vi "BL_TestConnection.vi"(8 "error in (no error)":errorcluster, 11 "Potentiostat Galvanostat in":refnum<class "Potentiostat Galvanostat.lvclass">) -> (0 "error out":errorcluster, 3 "Potentiostat Galvanostat out":refnum<class "Potentiostat Galvanostat.lvclass">)   [LabVIEW 2018, in "Potentiostat Galvanostat.lvclass"]
doc: "This function tests the communication with the selected instrument."
uses:
  Potentiostat Galvanostat.lvclass
  Potentiostat Galvanostat.lvclass/Potentiostat Galvanostat.ctl
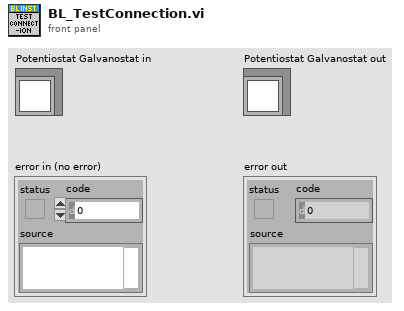
[diagram p1: front panel]
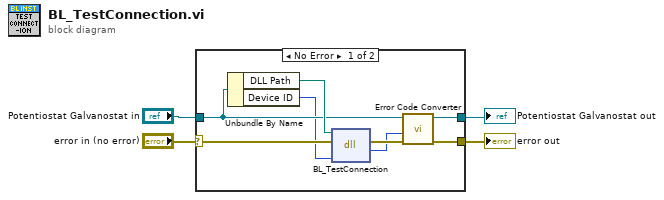
[diagram p0: block diagram]
diagram:
  n1 = case shown="No Error" "error in (no error)" {
    selector: "error in (no error)" -> [w11 w14]
    tunnel: [w9 w14] -> w3
    tunnel: [w8 w13] -> w1
    tunnel: "Potentiostat Galvanostat in" -> [w6 w13]
    frame No Error {
      n2 = Unbundle By Name(w6) -> ("DLL Path"=w12:path, "Device ID"=w5:i32)
      n3 = dll-call lib="C:/Projects/LabVIEW/BioLogic Instrument Driver/libs/EC-Lab Development Package/EClib.*" fn="BL_TestConnection"(path in=w12, error in=w11, "Device ID"=w5) -> (error out=w10:errorcluster, "Error Code"=w7:i32)  [unwired: 2 in, 1 out]
      n4 = call-dynamic "Error Code Converter.vi"("error in (no error)"=w10, "Error Code"=w7, "Potentiostat Galvanostat in"=w6) -> ("error out"=w9:errorcluster, "Potentiostat Galvanostat out"=w8:refnum<class "Potentiostat Galvanostat.lvclass">)  [unwired: 7 in]
    }
    frame Error {
    }
  }
  "error out" <- w3
  "Potentiostat Galvanostat out" <- w1
